vi "Bundle.vi"(9 "Boolean":bool, 10 "String":string, 11 "Numeric":dbl) -> (3 "output cluster":T1)   [LabVIEW 2024]
panel:
  in  "Cluster":T1
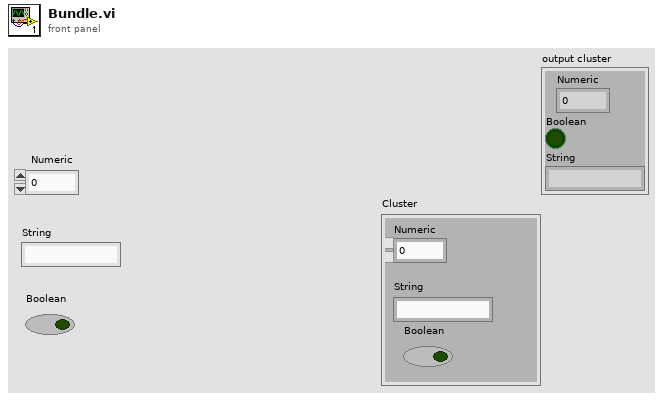
[diagram p1: front panel]
types:
  T1 = cluster{"Numeric":dbl, "Boolean":bool, "String":string}
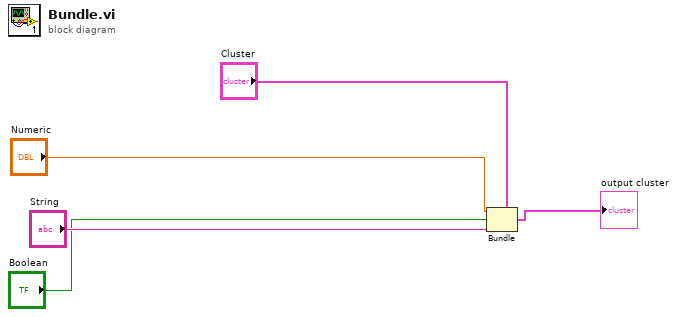
[diagram p0: block diagram]
diagram:
  n1 = Bundle(cluster="Cluster", "Numeric"="Numeric", "Boolean"="Boolean", "String"="String") -> (→"output cluster":T1)
